vi "ClientSrv Tag to Path.vi"(1 "tree tag":string) -> (0 "path":path)   [LabVIEW 2012]
doc: "Converts a tree tag surrounded by quotes into a path. Quotes are required because tree tags cannot hold strings that start or end with whitespace."
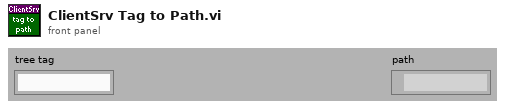
[diagram p1: front panel]
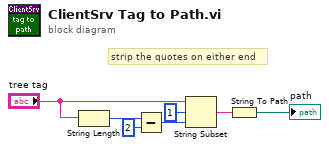
[diagram p0: block diagram]
diagram:
  # "strip the quotes on either end"
  n1 = String Length(string="tree tag") -> (length=w3:i32)
  n2 = Subtract(x=w3, y=2) -> (x-y=w4:i32)
  n3 = String Subset(string="tree tag", offset (0)=1, length (rest)=w4) -> (substring=w5:string)
  n4 = String To Path(string=w5) -> (path=→"path":path)
